vi "Get Set Collection Data Size.vi"(8 "error in (no error)":errorcluster, 10 "Data String":u8[](array[numeric]), 11 "Type Descriptor":i16[](array[numeric])) -> (0 "error out":errorcluster, 2 "Data Size":i32)   [LabVIEW 2017, in "Composition.lvlib"]
doc: "Gets the data size of a set collection."
uses:
  Composition.lvlib
  Get Data Type.vi/2a0888ac-0230-421b-a610-ddb651202d87.vi
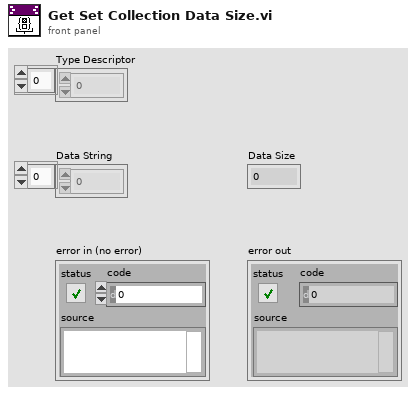
[diagram p1: front panel]
types:
  T1 = typedef "Composition.lvlib/Data Type.ctl" = enum16{"Void", "I8", "I16", "I32", "I64", "U8", "U16", "U32", "U64", "SGL", "DBL", "EXT", "CSG", "CDB", "CXT", "0x0F", "0x10", "0x11", "0x12", "0x13", "0x14", "Enum U8", "Enum U16", "Enum U32", "0x18", "SGL Physical", "DBL Physical", "EXT Physical", "CSG Physical", "CDB Physical", "CXT Physical", "0x1F", "Boolean U16", "Boolean U8", "0x22", "0x23", "0x24", "0x25", "0x26", "0x27", "0x28", "0x29", "0x2A", "0x2B", "0x2C", "0x2D", "0x2E", "0x2F", "String", "0x31", "Path", "Picture", "CString", "PString", "0x36", "Tag", "0x38", "0x39", "0x3A", "0x3B", "0x3C", "0x3D", "0x3E", "SubString", "Array", "Array Data Ptr", "0x42", "0x43", "0x44", "0x45", "0x46", "0x47", "0x48", "0x49", "0x4A", "0x4B", "0x4C", "0x4D", "0x4E", "SubArray", "Cluster", "0x51", "0x52", "Variant", "Waveform", "0x55", "0x56", "0x57", "0x58", "0x59", "0x5A", "0x5B", "0x5C", "0x5D", "CFX", "FXP", "Block", "Type Block", "Void Block", "Aligned Block", "Repeated Block", "Alignment Marker", "0x66", "0x67", "0x68", "0x69", "0x6A", "0x6B", "0x6C", "0x6D", "0x6E", "0x6F", "Refnum", "0x71", "0x72", "Set Collection", "Map Collection", "0x75", "0x76", "0x77", "0x78", "0x79", "0x7A", "0x7B", "0x7C", "0x7D", "0x7E", "0x7F", "Ptr", "0x81", "0x82", "Ptr to", "EXT Data", "0x85", "0x86", "0x87", "0x88", "0x89", "0x8A", "0x8B", "0x8C", "0x8D", "0x8E", "0x8F", "0x90", "0x91", "0x92", "0x93", "0x94", "0x95", "0x96", "0x97", "0x98", "0x99", "0x9A", "0x9B", "0x9C", "0x9D", "0x9E", "0x9F", "Array Interface", "Interface to Data", "0xA2", "0xA3", "0xA4", "0xA5", "0xA6", "0xA7", "0xA8", "0xA9", "0xAA", "0xAB", "0xAC", "0xAD", "0xAE", "0xAF", "0xB0", "0xB1", "0xB2", "0xB3", "0xB4", "0xB5", "0xB6", "0xB7", "0xB8", "0xB9", "0xBA", "0xBB", "0xBC", "0xBD", "0xBE", "0xBF", "0xC0", "0xC1", "0xC2", "0xC3", "0xC4", "0xC5", "0xC6", "0xC7", "0xC8", "0xC9", "0xCA", "0xCB", "0xCC", "0xCD", "0xCE", "0xCF", "0xD0", "0xD1", "0xD2", "0xD3", "0xD4", "0xD5", "0xD6", "0xD7", "0xD8", "0xD9", "0xDA", "0xDB", "0xDC", "0xDD", "0xDE", "0xDF", "0xE0", "0xE1", "0xE2", "0xE3", "0xE4", "0xE5", "0xE6", "0xE7", "0xE8", "0xE9", "0xEA", "0xEB", "0xEC", "0xED", "0xEE", "0xEF", "Function", "TypeDef", "PolyVI", "0xF3", "0xF4", "0xF5", "0xF6", "0xF7", "0xF8", "0xF9", "0xFA", "0xFB", "0xFC", "0xFD", "0xFE", "0xFF"}
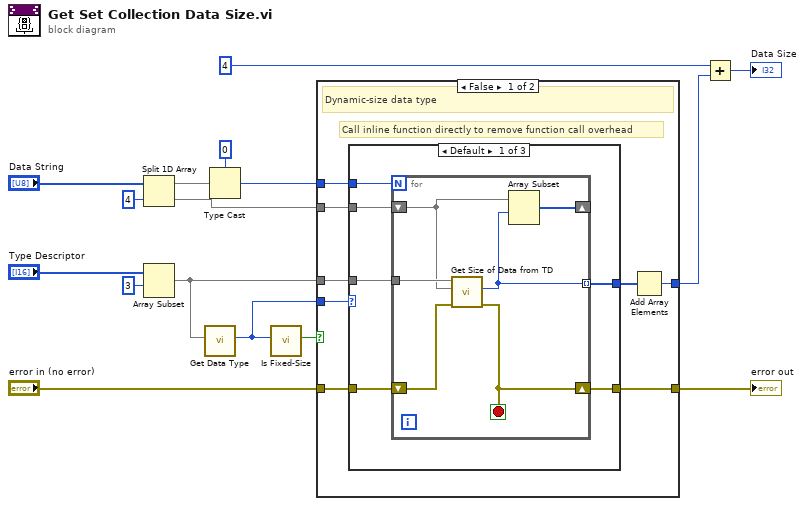
[diagram p0: block diagram]
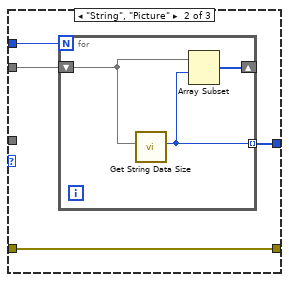
[diagram p2: hidden frame]
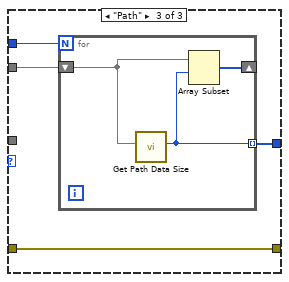
[diagram p3: hidden frame]
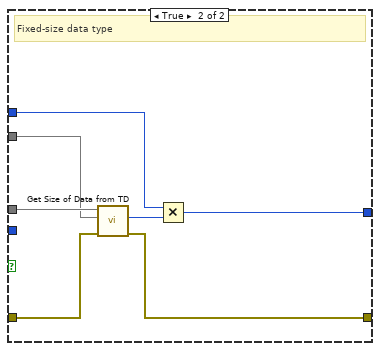
[diagram p4: hidden frame]
diagram:
  n1 = Split 1D Array(array="Data String", index=4) -> (first subarray=w12:u8[], second subarray=w15:u8[])
  n2 = Array Subset(array="Type Descriptor", index=3) -> (w8:i16[])  [unwired: 1 in]
  n3 = call "Get Data Type.vi"("Type Descriptor"=w8) -> ("Data Type"=w1:T1)  [unwired: 10 in]
  n4 = Type Cast(type=0, x=w12) -> (*(type *) &x=w10:i32)
  n5 = call "Is Fixed-Size.vi"("Data Type"=w1) -> ("Is Fixed-Size"=w7:bool)  [unwired: 10 in]
  n6 = case shown="False" w7 {
    tunnel: w15 -> [w24 w56]
    tunnel: w10 -> [w23 w53]
    tunnel: [w17 w54] -> w9
    tunnel: w8 -> [w22 w57]
    tunnel: "error in (no error)" -> [w21 w52]
    tunnel: [w20 w51] -> w3
    tunnel: w1 -> [w19 _]
    frame False {
      # "Call inline function directly to remove function call overhead"
      # "Dynamic-size data type"
      n7 = case shown="Default" w19 {
        tunnel: w24 -> [w30 w39 w46]
        tunnel: w23 -> [w29 w40 w47]
        tunnel: [w25 w37 w44] -> w18
        tunnel: w22 -> [w28 _ _]
        tunnel: w21 -> [w27 w38 w45]
        tunnel: [w26 w38 w45] -> w20
        frame Default {
          n8 = for {
            N: w29 -> [_]
            tunnel: w28 -> [w36]
            shift-right: [w34] -> _
            shift-left: w30 -> [w35]
            tunnel: [w33] -> w25 mode=indexing
            shift-right: [w31] -> w26
            shift-left: w27 -> [w32]
            stop <- w31 stop-if-true
            n9 = call "Get Size of Data from TD.vi"("error in (no error)"=w32, "Data String"=w35, "Type Descriptor"=w36) -> ("error out"=w31:errorcluster, "Size of Data"=w33:i32)  [unwired: 7 in]
            n10 = Array Subset(array=w35, index=w33) -> (w34:u8[])  [unwired: 1 in]
          }
        }
        frame "String", "Picture" {
          n11 = for {
            N: w40 -> [_]
            shift-right: [w43] -> _
            shift-left: w39 -> [w42]
            tunnel: [w41] -> w37 mode=indexing
            n12 = call "Get String Data Size.vi"("Data String"=w42) -> ("Data Size"=w41:i32)  [unwired: 10 in]
            n13 = Array Subset(array=w42, index=w41) -> (w43:u8[])  [unwired: 1 in]
          }
        }
        frame "Path" {
          n14 = for {
            N: w47 -> [_]
            shift-right: [w50] -> _
            shift-left: w46 -> [w49]
            tunnel: [w48] -> w44 mode=indexing
            n15 = call "Get Path Data Size.vi"("Data String"=w49) -> ("Data Size"=w48:i32)  [unwired: 10 in]
            n16 = Array Subset(array=w49, index=w48) -> (w50:u8[])  [unwired: 1 in]
          }
        }
      }
      n17 = Add Array Elements(numeric array=w18) -> (sum=w17:i32)
    }
    frame True {
      # "Fixed-size data type"
      n18 = call "Get Size of Data from TD.vi"("error in (no error)"=w52, "Data String"=w56, "Type Descriptor"=w57) -> ("error out"=w51:errorcluster, "Size of Data"=w55:i32)  [unwired: 7 in]
      n19 = Multiply(x=w53, y=w55) -> (x*y=w54:i32)
    }
  }
  "error out" <- w3
  n20 = Add(x=4 ("y"), y=w9) -> (x+y=→"Data Size":i32)
